vi "FRCts20_WebMethods_Request_PUT.vi"(7 "LabVIEW Web Service Request":refnum<class "Web Request.lvclass">, 10 "Action":string) -> ()   [LabVIEW 2014, in "FRCts20_WebMethods.lvlib"]
doc: "<B>PUT</B> on the specified <B>request</B> resource\n\n<B>Required XML Data : </B>\n<Request>\n <Status>[<B>Open</B>, <B>In Work</B>, <B>Closed</B>]</Status>\n</Request>\n\n<B>Required HTML Post Data : </B>\nStatus: [<B>Open</B>, <B>In Work</B>, <B>Closed</B>]\n\nhttp://<server address>:<port>/FRCts/request/<B>request</B>"
uses:
  FRCts20_WebMethods.lvlib
  <vilib>/wsapi/Web Request.lvclass
  Backend/source/VI Source/FRCts20_Backend_API/Notes.ctl
  Backend/source/VI Source/FRCts20_Backend_API/ApiReturn.ctl
  Backend/source/VI Source/FRCts20_Backend_API/NotesRoot.ctl
  Backend/source/VI Source/FRCts20_Backend_API/FRCts20_Backend_API_Command_Note.ctl
  Backend/source/VI Source/FRCts20_Backend_API/FRCts20_Backend_API_Comment.vi
  Backend/source/VI Source/FRCts20_Backend_API/FRCts20_Backend_API.lvlib
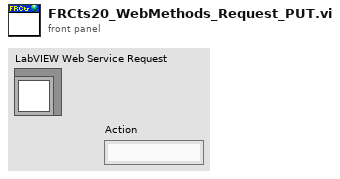
[diagram p1: front panel]
types:
  T1 = typedef "FRCts20_Backend_Engine.lvlib/FRCts20_Backend_API.lvlib/FRCts20_Backend_API_Command_Note.ctl" = string
  T2 = typedef "FRCts20_Backend_Engine.lvlib/FRCts20_Backend_API.lvlib/Notes.ctl" = cluster{"APIReturn":T3, "NotesRoot":T4}
  T3 = typedef "FRCts20_Backend_Engine.lvlib/FRCts20_Backend_API.lvlib/ApiReturn.ctl" = string
  T4 = typedef "FRCts20_Backend_Engine.lvlib/FRCts20_Backend_API.lvlib/NotesRoot.ctl" = cluster{"NoteIndex":u32, "ReqNumber":i32, "NoteText":string, "TimeEntered":string, "Author":string, "Solution":i32, "Deleted":i32}[]
  T5 = cluster{"NoteIndex":u32, "ReqNumber":i32, "NoteText":string, "TimeEntered":string, "Author":string, "Solution":i32, "Deleted":i32}
  T6 = cluster{"NoteIndex":u32, "ReqNumber":i32, "NoteText":string, "TimeEntered":string, "Author":string, "Solution":i32, "Deleted":i32}[]
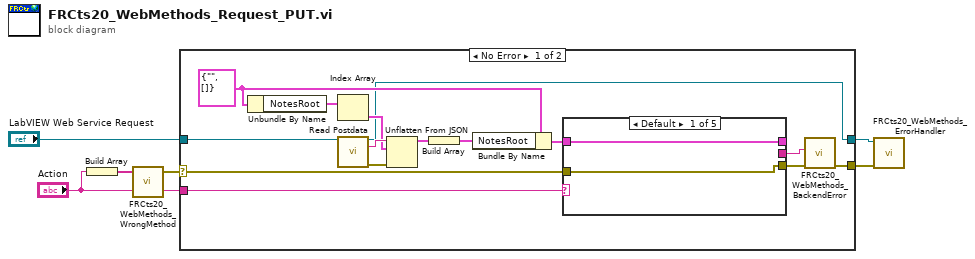
[diagram p0: block diagram]
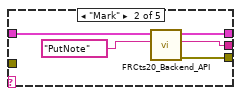
[diagram p2: hidden frame]
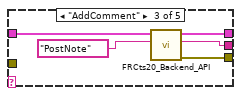
[diagram p3: hidden frame]
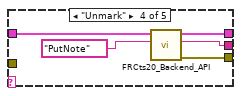
[diagram p4: hidden frame]
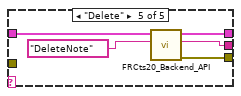
[diagram p5: hidden frame]
diagram:
  n1 = Build Array("Action") -> (w3:string[])
  n2 = call "FRCts20_WebMethods_WrongMethod.vi"("Method Inputs"=w3) -> ("error out"=w2:errorcluster)  [unwired: 4 in]
  n3 = case shown="No Error" w2 {
    selector: w2 -> [w20 w44]
    tunnel: [w8 w45] -> w6
    tunnel: [w7 w44] -> w5
    tunnel: "Action" -> [w21 _]
    tunnel: "LabVIEW Web Service Request" -> [w13 w45]
    frame No Error {
      w10 = T2 {"APIReturn"="", "NotesRoot"=[]} ("Note In")
      n4 = Unbundle By Name(w10) -> ("NotesRoot"=w17:T4)
      n5 = Index Array(array=w17) -> (element=w11:T5)  [unwired: 1 in]
      n6 = call <vilib>:"Read Postdata.vi"("LabVIEW Web Service Request"=w13) -> ("LabVIEW Web Service Request out"=w8:refnum<class "Web Request.lvclass">, "postdata"=w12:string, "error out"=w14:errorcluster)  [unwired: 12 in]
      n7 = Unflatten From JSON(JSON string=w12, type and defaults=w11, error in (no error)=w14) -> (value=w15:T5)  [unwired: 4 in, 1 out]
      n8 = Build Array(w15) -> (w16:T6)
      n9 = Bundle By Name(cluster=w10, "NotesRoot"=w16) -> (w9:T2)
      n10 = case shown="Default" w21 {
        tunnel: [w22 w26 w33 w37 w40] -> _
        tunnel: [w23 w28 w32 w38 w43] -> w19
        tunnel: w20 -> [w23 _ _ _ _]
        tunnel: [_ w27 w31 w36 w42] -> w18
        tunnel: w9 -> [w22 w25 w30 w35 w41]
        frame Default {
        }
        frame "Mark" {
          n11 = call-poly "FRCts20_Backend_API.vi"("Command"=T1 "PutNote", "Note In"=w25) -> ("error out"=w28:errorcluster, "Status"=w27:string, "Note Out"=w26:T2)  [unwired: 7 in]
        }
        frame "AddComment" {
          n12 = call-poly "FRCts20_Backend_API.vi"("Command"=T1 "PostNote", "Note In"=w30) -> ("error out"=w32:errorcluster, "Status"=w31:string, "Note Out"=w33:T2)  [unwired: 7 in]
        }
        frame "Unmark" {
          n13 = call-poly "FRCts20_Backend_API.vi"("Command"=T1 "PutNote", "Note In"=w35) -> ("error out"=w38:errorcluster, "Status"=w36:string, "Note Out"=w37:T2)  [unwired: 7 in]
        }
        frame "Delete" {
          n14 = call-poly "FRCts20_Backend_API.vi"("Command"=T1 "DeleteNote", "Note In"=w41) -> ("error out"=w43:errorcluster, "Status"=w42:string, "Note Out"=w40:T2)  [unwired: 7 in]
        }
      }
      n15 = call "FRCts20_WebMethods_BackendError.vi"("error in (no error)"=w19, "Status"=w18) -> ("error out"=w7:errorcluster)  [unwired: 8 in, 1 out]
    }
    frame Error {
    }
  }
  n16 = call "FRCts20_WebMethods_ErrorHandler.vi"("error in"=w5, "LabVIEW Web Service Request"=w6) -> ()  [unwired: 8 in, 2 out]
